vi "tcs_issueCommand_target.vi"(8 "error in (no error)":errorcluster, 11 "command_target_Ctl":T1={"targetId"=0, "fieldId"=0, "groupId"=0, "filter"="                                                                ", "requestTime"=0.0, "ra"=0.0, "dec"=0.0, "angle"=0.0, "num_exposures"=0, "exposure_times"=0, "slew_time"=0.0}) -> (0 "error out":errorcluster, 2 "function return":i32, 3 "command_target_Ctl out":T1={"targetId"=0, "fieldId"=0, "groupId"=0, "filter"="                                                                ", "requestTime"=0.0, "ra"=0.0, "dec"=0.0, "angle"=0.0, "num_exposures"=0, "exposure_times"=0, "slew_time"=0.0})   [LabVIEW 2016, in "SALLV_tcs.lvlib"]
doc: "int tcs_shm_issueCommand_targetLV(tcs_command_targetLV *command_target_Ctl );"
uses:
  SALLV_tcs.lvlib
  DataTypes/command_target.ctl
  SALLV_tcs.so
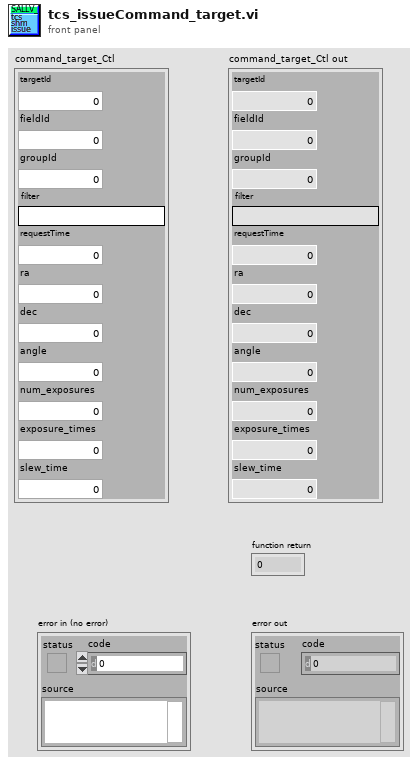
[diagram p1: front panel]
types:
  T1 = typedef "SALLV_tcs.lvlib/command_target.ctl" = cluster{"targetId":i32, "fieldId":i32, "groupId":i32, "filter":string, "requestTime":dbl, "ra":dbl, "dec":dbl, "angle":dbl, "num_exposures":i32, "exposure_times":i32, "slew_time":dbl}
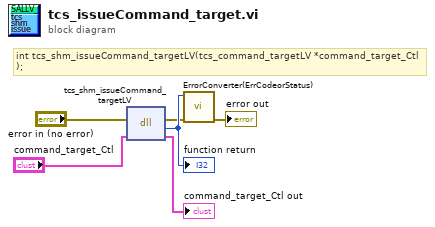
[diagram p0: block diagram]
diagram:
  # "int tcs_shm_issueCommand_targetLV(tcs_command_targetLV *command_target_Ctl );"
  n1 = dll-call lib="home/andres/Desktop/SALLV_tcs/SALLV_tcs.*" fn="tcs_shm_issueCommand_targetLV"(error in="error in (no error)", "command_target_Ctl"="command_target_Ctl") -> (error out=w2:errorcluster, w6:i32, "command_target_Ctl"=→"command_target_Ctl out":T1)  [unwired: 2 in, 1 out]
  "function return" <- w6
  n2 = call "ErrorConverter(ErrCodeorStatus).vi"("error in (no error)"=w2, "error code"=w6) -> ("error out"=→"error out":errorcluster)  [unwired: 9 in]
